vi "Save_VI.vi"(9 "save press as image":bool, 10 "save pressure as excel":bool, 11 "XYGraph in":refnum<vi>) -> ()   [LabVIEW 2017]
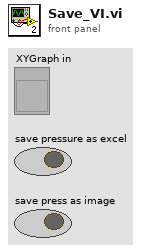
[diagram p1: front panel]
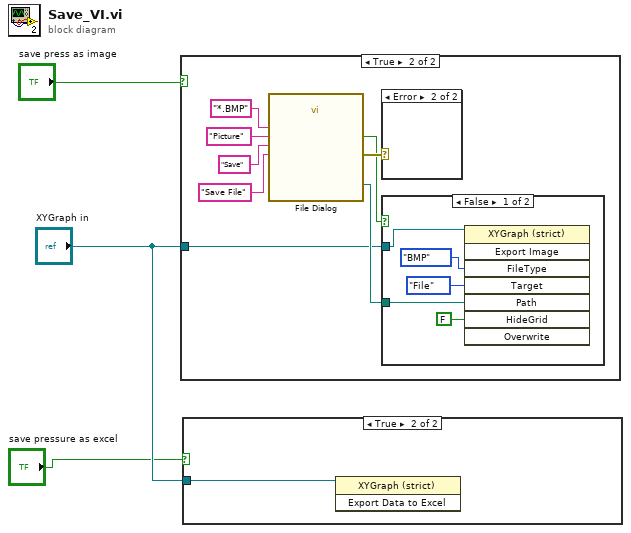
[diagram p0: block diagram]
diagram:
  n1 = case shown="True" "save press as image" {
    tunnel: "XYGraph in" -> [_ w4]
    frame False {
    }
    frame True {
      n2 = call "File Dialog"("prompt"="Save File", "button label"="Save", "pattern (all files)"="*.BMP", "pattern label"="Picture") -> ("selected path"=w6:path, "cancelled"=w5:bool, "error out"=w7:errorcluster)  [unwired: 8 in, 1 out]
      n3 = case shown="Error" w7 {
        frame No Error {
        }
        frame Error {
        }
      }
      n4 = case shown="False" w5 {
        tunnel: w6 -> [w14 _]
        tunnel: w4 -> [w12 _]
        frame False {
          n5 = invoke on="Invoke Node" class="XYGraph (strict)" method="Export Image"(reference=w12, "FileType"=enum32{"BMP", "EPS", "EMF", "PICT"}."BMP" ("File Type"), "Target"=enum32{"File", "Clipboard"}."File", "Path"=w14, "HideGrid"=FALSE ("Hide Grid")) -> ()  [unwired: 3 in, 8 out]
        }
        frame True {
        }
      }
    }
  }
  n6 = case shown="True" "save pressure as excel" {
    tunnel: "XYGraph in" -> [_ w17]
    frame False {
    }
    frame True {
      n7 = invoke on="Invoke Node" class="XYGraph (strict)" method="Export Data to Excel"(reference=w17) -> ()  [unwired: 2 in, 3 out]
    }
  }
